vi "VSI Write Bytes.vi"(6 "Len":u16, 7 "pWriteData":u8[](array[numeric])=array[10240 elements], 9 "SPIIndex":i32, 10 "DevIndex":i32, 11 "DevType":i32) -> (3 "function return":i32)   [LabVIEW 2010, in "ControlSPI.lvlib"]
doc: "int WINAPI VSI_WriteBytes(int DevType,int DevIndex,int SPIIndex,unsigned char *pWriteData,unsigned short Len);"
uses:
  ControlSPI.lvlib
  ControlSPI/Ginkgo_Driver.dll
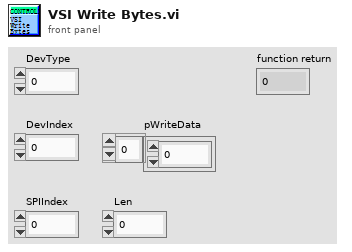
[diagram p1: front panel]
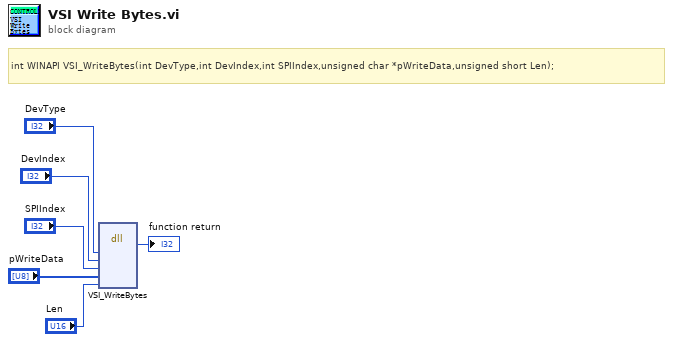
[diagram p0: block diagram]
diagram:
  # "int WINAPI VSI_WriteBytes(int DevType,int DevIndex,int SPIIndex,unsigned char *pWriteData,unsigned short Len);"
  n1 = dll-call lib="E:/Project/vt_ginkgo/truck/Ginkgo Driver/vs2010/Ginkgo_USB-I2C&SPI&CAN_API_v2.0.3.3/lib/labview_32bit/ControlSPI/Ginkgo_Driver.*" fn="VSI_WriteBytes"("DevType"="DevType", "DevIndex"="DevIndex", "SPIIndex"="SPIIndex", "pWriteData"="pWriteData", "Len"="Len") -> (→"function return":i32)  [unwired: 8 in, 2 out]
